vi "testPDO.vi"() -> ()   [LabVIEW 2014]
uses:
  <vilib>/CANopenLib/CANOPEN.llb/CANopen BaudRate.ctl
  <vilib>/CANopenLib/CANOPEN.llb/CANopen Interface Create.vi
  <vilib>/CANopenLib/CANOPEN.llb/CANopen RPDO Create.vi
  <vilib>/CANopenLib/CANOPEN.llb/CANopen Convert To Data [U16].vi
  <vilib>/CANopenLib/CANOPEN.llb/CANopen RPDO Close.vi
  <vilib>/CANopenLib/CANOPEN.llb/CANopen Interface Close.vi
panel:
  in  "baud rate":T1 items=["1 Mbit/s"=0, "800 kbit/s"=1, "500 kbit/s"=2, "250 kbit/s"=3, "125 kbit/s"=4, "50 kbit/s"=6, "20 kbit/s"=7, "10 kbit/s"=8]
  in  "interface name":u32(ring) items=["CANopen01", "CANopen02", "CANopen03", "CANopen04", "CANopen05", "CANopen06", "CANopen07", "CANopen08", "CANopen09", "CANopen10", "CANopen11", "CANopen12", "CANopen13", "CANopen14", "CANopen15", "CANopen16", "CANopen17", "CANopen18", "CANopen19", "CANopen20", "CANopen21", "CANopen22", "CANopen23", "CANopen24", "CANopen25", "CANopen26", "CANopen27", "CANopen28", "CANopen29", "CANopen30", "CANopen31", "CANopen32"]
  out "error out":errorcluster caption="Fehler (Ausgang)"
  in  "error in (no error)":errorcluster caption="Fehler (Eingang, kein Fehler)"
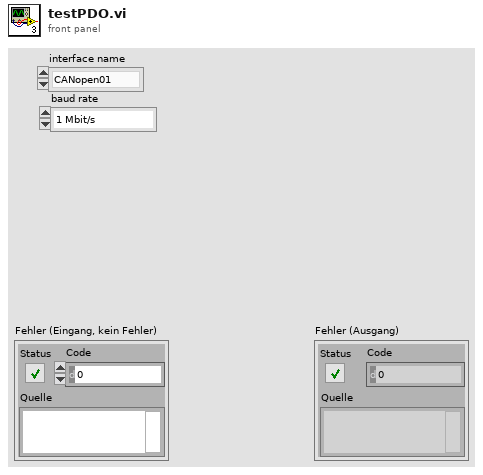
[diagram p1: front panel]
types:
  T1 = typedef "CANopen BaudRate.ctl" = u32
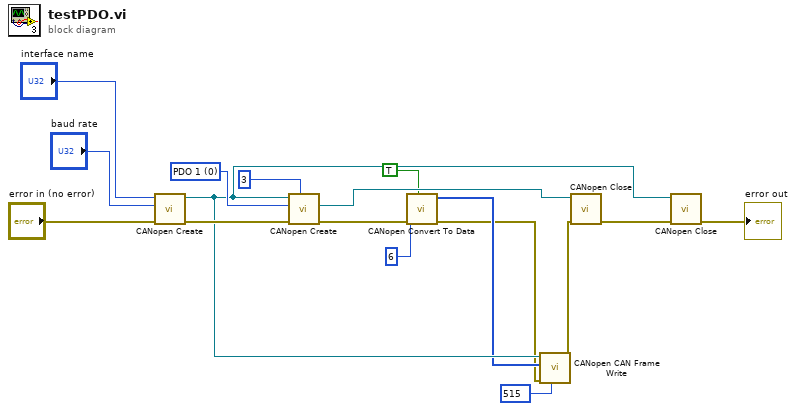
[diagram p0: block diagram]
diagram:
  w12 = u8 0 items=["PDO 1", "PDO 2", "PDO 3", "PDO 4"] ("PDO channel")
  n1 = call-poly <vilib>:"CANopen Create.vi"("error in (no error)"="error in (no error)", "baud rate"="baud rate", "interface name"="interface name") -> ("error out"=w17:errorcluster, "interface object out"=w5:refnum<k20>)  [unwired: 7 in]
  n2 = call-poly <vilib>:"CANopen Create.vi"("node-ID"=u8 3, "error in (no error)"=w17, "PDO channel"=w12, "interface object in"=w5) -> ("error out"=w8:errorcluster, "RPDO object out"=w11:refnum<k20>)  [unwired: 5 in, 1 out]
  n3 = call-poly <vilib>:"CANopen Convert To Data.vi"("trim"=TRUE, "error in (no error)"=w8, "unsigned 16-bit integer"=u16 6) -> ("error out"=w1:errorcluster, "CANopen data out"=w4:u8[])  [unwired: 7 in]
  n4 = call <vilib>:"CANopen CAN Frame Write.vi"("COB-ID (0)"=u32 515, "error in (no error)"=w1, "CAN message data"=w4, "interface object  in"=w5) -> ("error out"=w3:errorcluster)  [unwired: 6 in, 1 out]
  n5 = call-poly <vilib>:"CANopen Close.vi"("error in (no error)"=w3, "RPDO object in"=w11) -> ("error out"=w10:errorcluster)  [unwired: 9 in]
  n6 = call-poly <vilib>:"CANopen Close.vi"("error in (no error)"=w10, "interface object in"=w5) -> ("error out"=→"error out":errorcluster)  [unwired: 9 in]
